vi "Database.SimpleWriteStationValues.vi"(8 "error in":errorcluster, 10 "FileName":string, 11 "Data in":T1 {"Variant"."TS"."TV"."minimum" format="%#.3f"; "Variant"."TS"."TV"."maximum" format="%#.3f"; "Variant"."TS"."TP"."value" format="%#.3f"}) -> (0 "error out":errorcluster, 3 "Data out":T1 {"Variant"."TS"."TV"."minimum" format="%#.3f"; "Variant"."TS"."TV"."maximum" format="%#.3f"; "Variant"."TS"."TP"."value" format="%#.3f"})   [LabVIEW 2016]
doc: "Write test results (measurement values) to proda database\n\nWabco 2017 All right reserved\nAuthor: maciej.szupienko@wabco-auto.com"
uses:
  Global/ApplicationGlobal.vi
  Database.Main.Data.Sets.ctl
  Database.Main.Data.Status.ctl
  ProdaNG/Controls/ProdaNG.ProcessResult.ctl
  ProdaNG/Controls/ProdaNG.ProcessStepResult.ctl
  ProdaNG/Controls/ProdaNG.TestStepResult.ctl
  ProdaNG/Controls/ProdaNG.TestValueResult.ctl
  ProdaNG/Controls/ProdaNG.Identification.ctl
  Database.Main.Data.ctl
  Database.Main.Data.Results.ctl
  ProdaNG/Controls/ProdaNG.TestStepParam.ctl
  ProdaNG/Controls/ProdaNG.TestValue.ctl
  ProdaNG/Controls/ProdaNG.TestStep.ctl
  ProdaNG/Controls/ProdaNG.ProcessStepParam.ctl
  Database.Main.Data.Variant.ctl
panel:
  out "Prod saved":bool
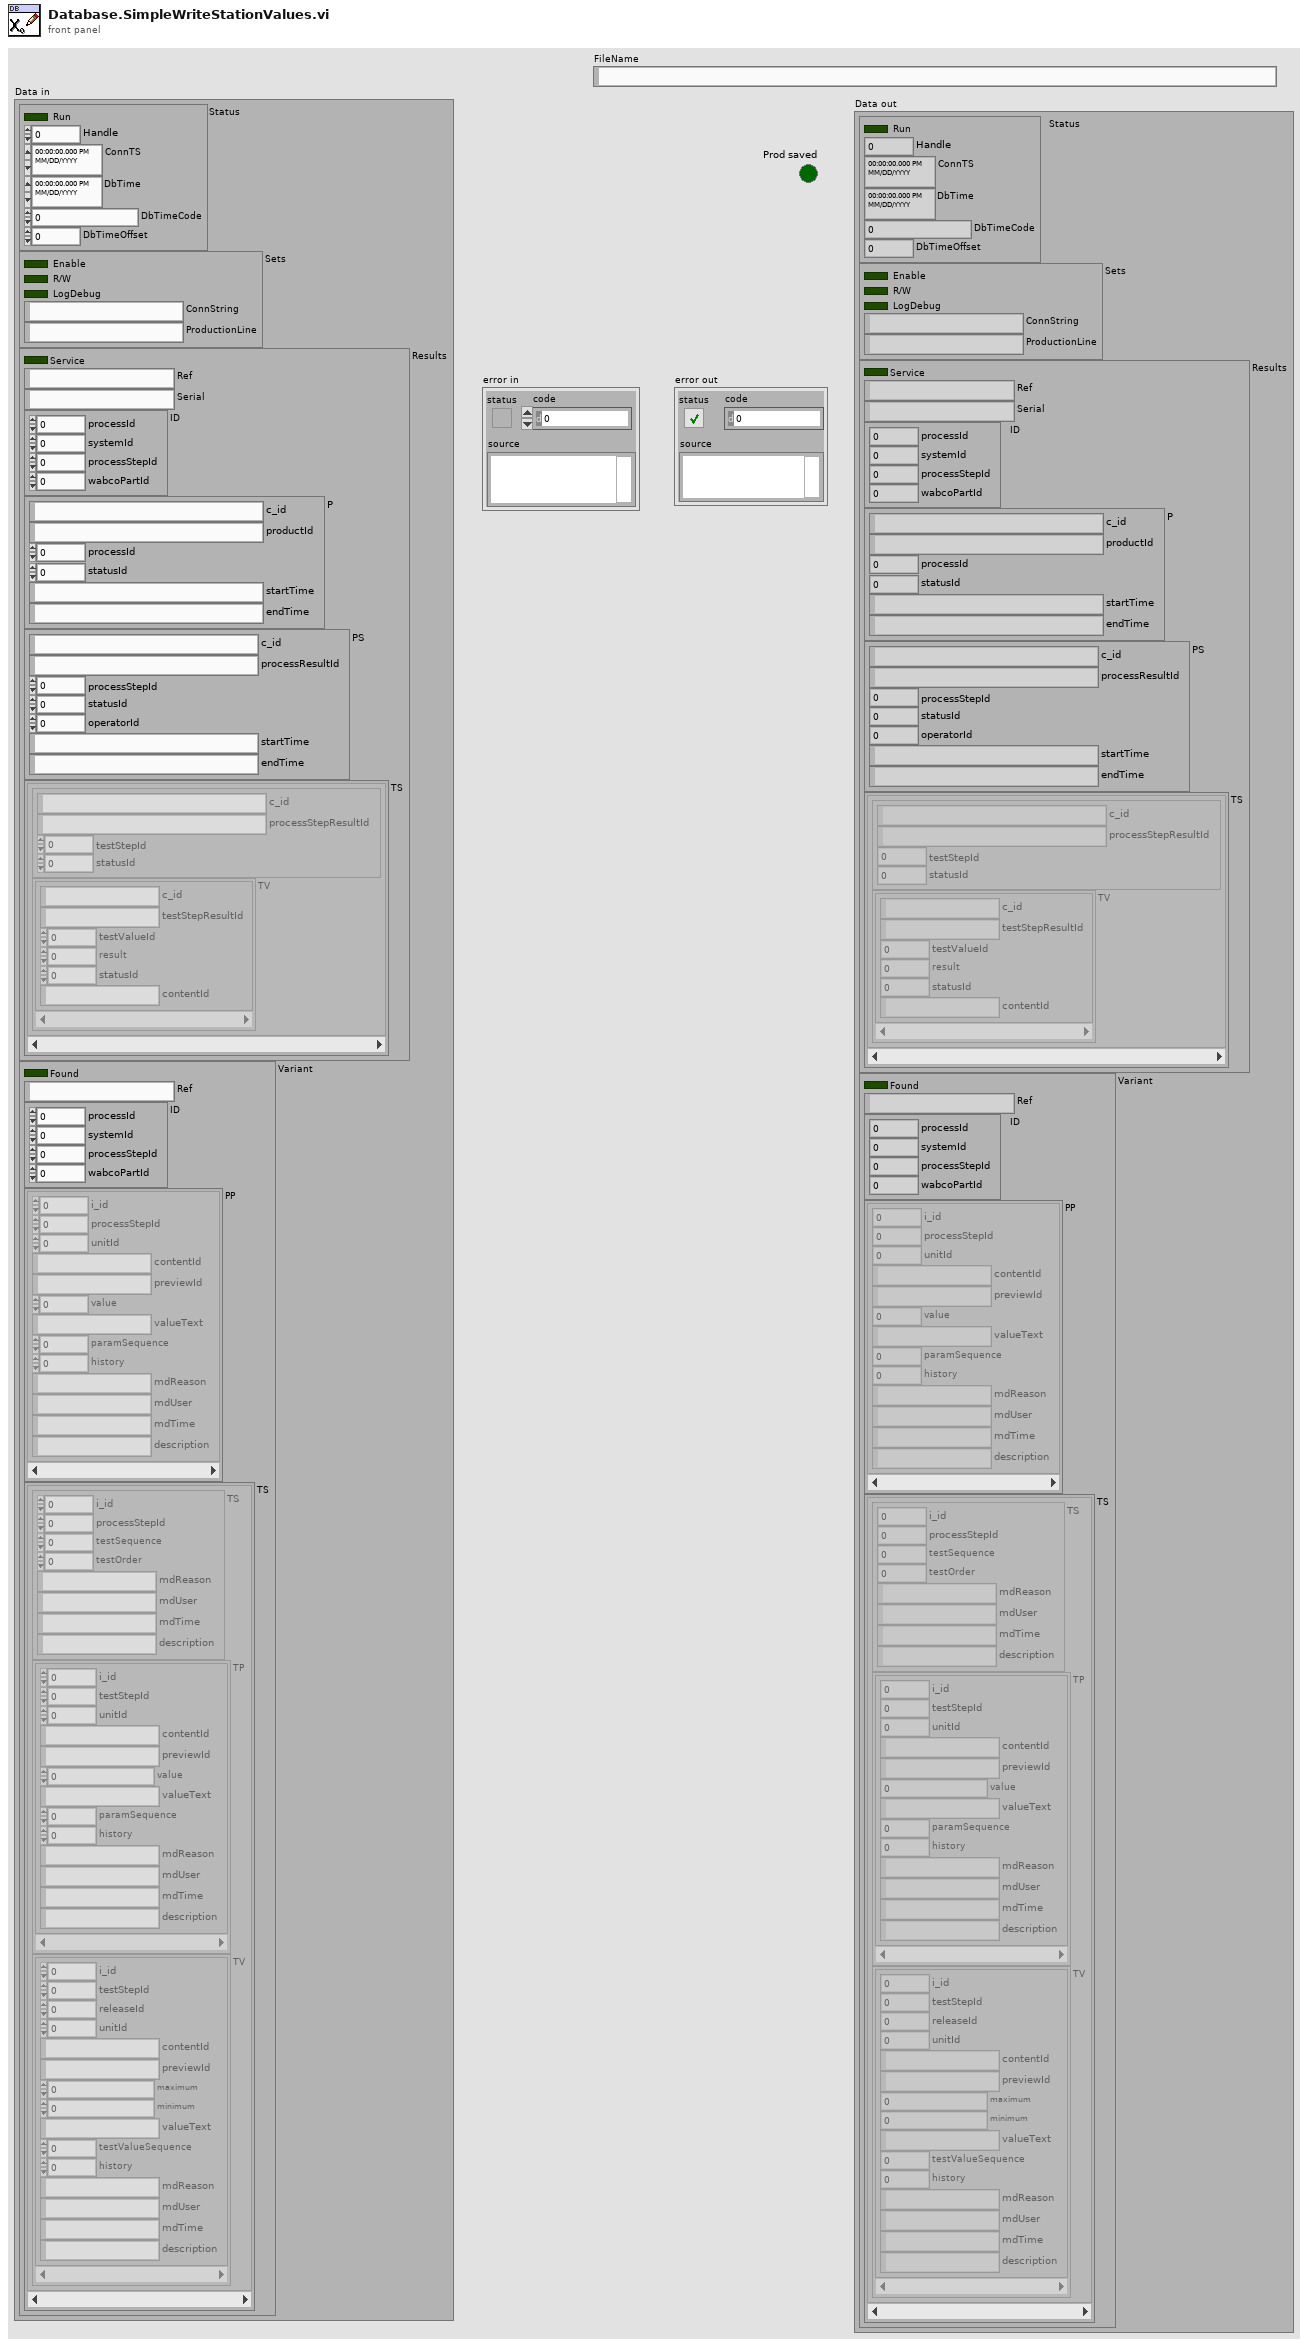
[diagram p1: front panel]
types:
  T1 = typedef "Database.Main.Data.ctl" = cluster{"Status":T2, "Sets":T3, "Results":T4, "Variant":T10}
  T2 = typedef "Database.Main.Data.Status.ctl" = cluster{"Run":bool, "Handle":i32, "ConnTS":timestamp, "DbTime":timestamp, "DbTimeCode":dbl, "DbTimeOffset":dbl}
  T3 = typedef "Database.Main.Data.Sets.ctl" = cluster{"Enable":bool, "R/W":bool, "LogDebug":bool, "ConnString":string, "ProductionLine":string}
  T4 = typedef "Database.Main.Data.Results.ctl" = cluster{"Service":bool, "Ref":string, "Serial":string, "ID":T5, "P":T6, "PS":T7, "TS":cluster{"TS":T8, "TV":T9[]}[]}
  T5 = typedef "ProdaNG.Identification.ctl" = cluster{"processId":i32, "systemId":i32, "processStepId":i32, "wabcoPartId":i32}
  T6 = typedef "ProdaNG.ProcessResult.ctl" = cluster{"c_id":string, "productId":string, "processId":i32, "statusId":i32, "startTime":string, "endTime":string}
  T7 = typedef "ProdaNG.ProcessStepResult.ctl" = cluster{"c_id":string, "processResultId":string, "processStepId":i32, "statusId":i32, "operatorId":i32, "startTime":string, "endTime":string}
  T8 = typedef "ProdaNG.TestStepResult.ctl" = cluster{"c_id":string, "processStepResultId":string, "testStepId":i32, "statusId":i32}
  T9 = typedef "ProdaNG.TestValueResult.ctl" = cluster{"c_id":string, "testStepResultId":string, "testValueId":i32, "result":dbl, "statusId":i32, "contentId":string}
  T10 = typedef "Database.Main.Data.Variant.ctl" = cluster{"Found":bool, "Ref":string, "ID":T5, "PP":T11[], "TS":cluster{"TS":T12, "TP":T13[], "TV":T14[]}[]}
  T11 = typedef "ProdaNG.ProcessStepParam.ctl" = cluster{"i_id":i32, "processStepId":i32, "unitId":i32, "contentId":string, "previewId":string, "value":dbl, "valueText":string, "paramSequence":i32, "history":i32, "mdReason":string, "mdUser":string, "mdTime":string, "description":string}
  T12 = typedef "ProdaNG.TestStep.ctl" = cluster{"i_id":i32, "processStepId":i32, "testSequence":i32, "testOrder":i32, "mdReason":string, "mdUser":string, "mdTime":string, "description":string}
  T13 = typedef "ProdaNG.TestStepParam.ctl" = cluster{"i_id":i32, "testStepId":i32, "unitId":i32, "contentId":string, "previewId":string, "value":dbl, "valueText":string, "paramSequence":i32, "history":i32, "mdReason":string, "mdUser":string, "mdTime":string, "description":string}
  T14 = typedef "ProdaNG.TestValue.ctl" = cluster{"i_id":i32, "testStepId":i32, "releaseId":i32, "unitId":i32, "contentId":string, "previewId":string, "maximum":dbl, "minimum":dbl, "valueText":string, "testValueSequence":i32, "history":i32, "mdReason":string, "mdUser":string, "mdTime":string, "description":string}
  T15 = typedef "ProdaNG.Product.ctl" = cluster{"c_id":string, "wabcoPartId":i32, "serialNumber":string, "comment":string, "individual":i32, "crProcessStepId":i32, "mdProcessStepId":i32, "crTime":string, "mdTime":string}
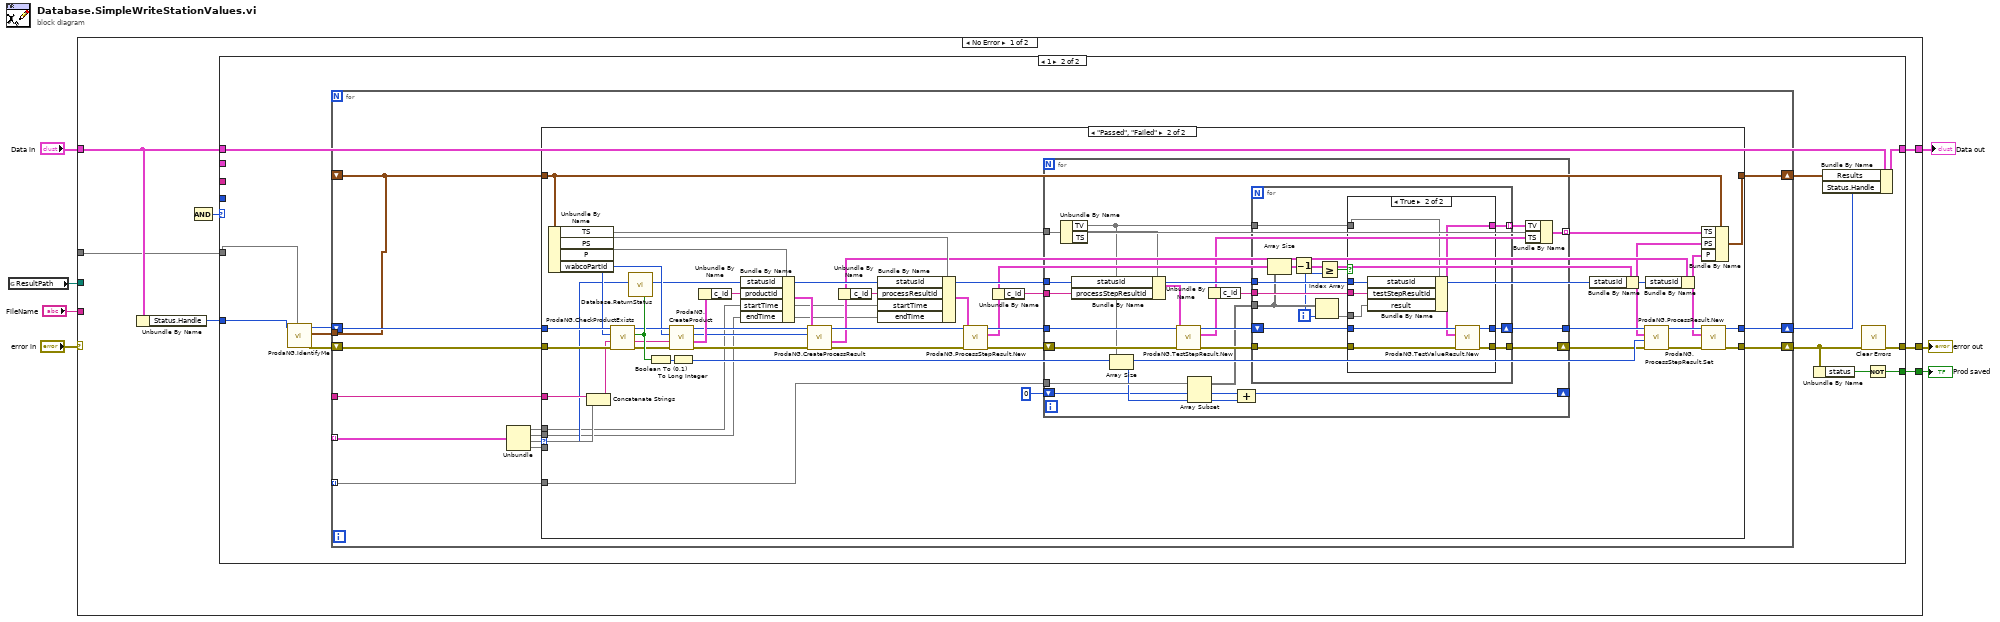
[diagram p0: block diagram]
diagram:
  n1 = global read "ApplicationGlobal.vi" "ResultPath"() -> (w3:path)
  n2 = case shown="No Error" "error in" {
    selector: "error in" -> [_ w146]
    tunnel: [w15 w146] -> w8
    tunnel: "Data in" -> [w11 w145]
    tunnel: [w16 w145] -> w5
    tunnel: [w14 _] -> w4
    tunnel: w3 -> [_ _]
    tunnel: "FileName" -> [_ _]
    tunnel: [w9 _] -> w1
    frame No Error {
      n3 = Unbundle By Name(w11) -> ("Status.Handle"=w10:i32)
      n4 = Compound Arithmetic op=AND() -> (w13:i32)  [unwired: 2 in]
      n5 = case shown="1" w13 {
        tunnel: [_ w36] -> w12
        tunnel: [_ w35] -> w17
        tunnel: w11 -> [w18 w34]
        tunnel: [w18 w33] -> w16
        tunnel: _ -> [_ w32]
        tunnel: [w19 w26] -> w15
        tunnel: [_ w27] -> w14
        tunnel: w10 -> [_ w23]
        tunnel: w9 -> [_ w22]
        frame 0, Default {
        }
        frame 1 {
          n6 = call "ProdaNG.IdentifyMe.vi"("systemName"=w22, "dbHandleIn"=w23) -> ("error out"=w21:errorcluster, "Identification"=w20:T5, "dbHandle"=w24:i32)  [unwired: 7 in]
          n7 = for {
            shift-right: [w45] -> w29
            shift-left: w21 -> [w49]
            shift-right: [w46] -> w30
            shift-left: w24 -> [w48]
            shift-right: [w47] -> w31
            shift-left: [w37] -> _
            tunnel: [w43] -> w25
            tunnel: _ -> [w44] mode=indexing
            tunnel: _ -> [w42] mode=indexing
            tunnel: w20 -> [w37]
            n8 = Unbundle(w44) -> ("date/time string"=w39, "date/time string"=w40, "StatusB"=w38, "SerialB"=w41)
            n9 = case shown="\"Passed\", \"Failed\"" w38 {
              selector: w38 -> [_ w57]
              tunnel: w49 -> [w52 w77]
              tunnel: w48 -> [w51 w76]
              tunnel: [w50 w67] -> w47
              tunnel: [w51 w63] -> w46
              tunnel: w37 -> [w50 w62]
              tunnel: [w52 w61] -> w45
              tunnel: w43 -> [_ w59]
              tunnel: w41 -> [_ w58]
              tunnel: w42 -> [_ w56]
              tunnel: w40 -> [_ w54]
              tunnel: w39 -> [_ w55]
              frame Default {
              }
              frame "Passed", "Failed" {
                n10 = Unbundle By Name(w62) -> ("TS"=w74, "PS"=w73, "P"=w72, "wabcoPartId"=w71:i32)
                n11 = Concatenate Strings(w59, w58) -> (w53:string)
                n12 = call "ProdaNG.CheckProductExists.vi"("error in (no error)"=w77, "serialNumber"=w53, "ID"=w71, "dbHandle"=w76) -> ("error out"=w79:errorcluster, "Results exist?"=w97:bool, "dbHandle out"=w75:i32)  [unwired: 2 in, 3 out]
                n13 = call "Database.ReturnStatus.vi"("repeat"=w97, "Status"=w57) -> ("Step.statusId"=w70:i32)  [unwired: 8 in, 1 out]
                n14 = Boolean To (0,1)(Boolean=w97) -> (0, 1=w78:i16)
                n15 = call "ProdaNG.CreateProduct.vi"("error in (no error)"=w79, "serialNumber"=w53, "ID"=w71, "dbHandle"=w75) -> ("error out"=w91:errorcluster, "Product out"=w96:T15, "dbHandle out"=w92:i32)  [unwired: 4 in, 1 out]
                n16 = To Long Integer(number=w78) -> (32bit integer=w95:i32)
                n17 = Unbundle By Name(w96) -> ("c_id"=w82:string)
                n18 = Bundle By Name(cluster=w72, "statusId"=w70, "productId"=w82, "startTime"=w55, "endTime"=w54) -> (w90:cluster{})
                n19 = call "ProdaNG.CreateProcessResult.vi"("error in (no error)"=w91, "ProcessResult"=w90, "ID"=w71, "dbHandle"=w92) -> ("error out"=w93:errorcluster, "ProcessResult 2"=w68:T6, "dbHandle out"=w94:i32)  [unwired: 5 in]
                n20 = Unbundle By Name(w68) -> ("c_id"=w83:string)
                n21 = Bundle By Name(cluster=w73, "statusId"=w70, "processResultId"=w83, "startTime"=w55, "endTime"=w54) -> (w89:cluster{})
                n22 = call "ProdaNG.ProcessStepResult.New.vi"("error in (no error)"=w93, "ProcessStepResult"=w89, "dbHandle"=w94) -> ("error out"=w81:errorcluster, "ProcessStepResult out"=w65:T7, "dbHandle"=w80:i32)  [unwired: 6 in]
                n23 = Unbundle By Name(w65) -> ("c_id"=w84:string)
                n24 = for {
                  tunnel: [w117] -> w86
                  tunnel: w84 -> [w115]
                  tunnel: w80 -> [w113]
                  tunnel: w56 -> [w103]
                  tunnel: w74 -> [w108]
                  tunnel: w70 -> [w109]
                  tunnel: [w104] -> w69 mode=indexing
                  shift-right: [w116] -> w85
                  shift-left: w81 -> [w114]
                  shift-right: [w98] -> _
                  shift-left: 0 -> [w100]
                  n25 = Unbundle By Name(w108) -> ("TV"=w102, "TS"=w106)
                  n26 = Bundle By Name(cluster=w106, "statusId"=w109, "processStepResultId"=w115) -> (w118:cluster{})
                  n27 = Array Size(array=w102) -> (size(s)=w101:i32)
                  n28 = call "ProdaNG.TestStepResult.New.vi"("error in (no error)"=w114, "TestStepResult"=w118, "dbHandle"=w113) -> ("error out"=w110:errorcluster, "TestStepResult out"=w105:T8, "dbHandle"=w111:i32)  [unwired: 6 in]
                  n29 = Array Subset(array=w103, index=w100, length=w101) -> (w99:void[])
                  n30 = Unbundle By Name(w105) -> ("c_id"=w112:string)
                  n31 = Compound Arithmetic op=ADD(w100, w101) -> (w98:i32)
                  n32 = for "results" {
                    tunnel: w110 -> [w132]
                    tunnel: [w129] -> w116
                    tunnel: w112 -> [w130]
                    shift-right: [w128] -> w117
                    shift-left: w111 -> [w131]
                    tunnel: w99 -> [w123]
                    tunnel: w109 -> [w127]
                    tunnel: w102 -> [w126]
                    tunnel: [w125] -> w107 mode=indexing
                    i -> [w121]
                    n33 = Array Size(array=w123) -> (size(s)=w120:i32)
                    n34 = Decrement(x=w120) -> (x-1=w119:i32)
                    n35 = Index Array(array=w123, index=w121) -> (element=w124)
                    n36 = Greater Or Equal?(x=w119, y=w121) -> (x >= y?=w122:bool)
                    n37 = case shown="True" w122 {
                      tunnel: w132 -> [w134 w144]
                      tunnel: w131 -> [w133 w143]
                      tunnel: w130 -> [_ w142]
                      tunnel: [w134 w141] -> w129
                      tunnel: [w133 w140] -> w128
                      tunnel: w127 -> [_ w139]
                      tunnel: w126 -> [w135 w138]
                      tunnel: [w135 w137] -> w125
                      tunnel: w124 -> [_ w136]
                      frame False {
                      }
                      frame True {
                        n38 = Bundle By Name(cluster=w138, "statusId"=w139, "testStepResultId"=w142, "result"=w136) -> (w137:cluster{})
                        n39 = call "ProdaNG.TestValueResult.New.vi"("error in (no error)"=w144, "TestValueResult"=w137, "dbHandle"=w143) -> ("error out"=w141:errorcluster, "dbHandle"=w140:i32)  [unwired: 7 in]
                      }
                    }
                  }
                  n40 = Bundle By Name(cluster=w108, "TV"=w107, "TS"=w105) -> (w104:cluster{})
                }
                n41 = Bundle By Name(cluster=w65, "statusId"=w70) -> (w64:T7)
                n42 = call "ProdaNG.ProcessStepResult.Set.vi"("error in (no error)"=w85, "isRepeat (0)"=w95, "ProcessStepResult"=w64, "dbHandle"=w86) -> ("error out"=w88:errorcluster, "dbHandle"=w87:i32)  [unwired: 6 in]
                n43 = Bundle By Name(cluster=w68, "statusId"=w70) -> (w66:T6)
                n44 = Bundle By Name(cluster=w62, "TS"=w69, "PS"=w64, "P"=w66) -> (w67:T5)
                n45 = call "ProdaNG.ProcessResult.New.vi"("error in (no error)"=w88, "ProcessResult"=w66, "dbHandle"=w87) -> ("error out"=w61:errorcluster, "dbHandle"=w63:i32)  [unwired: 6 in, 1 out]
              }
            }
          }
          n46 = Unbundle By Name(w29) -> ("status"=w28:bool)
          n47 = Bundle By Name(cluster=w34, "Results"=w31, "Status.Handle"=w30) -> (w33:T1)
          n48 = call <vilib>:"Clear Errors.vi"("error in (no error)"=w29) -> ("error out"=w26:errorcluster)  [unwired: 5 in, 1 out]
          n49 = Not(x=w28) -> (.not. x?=w27:bool)
        }
      }
    }
    frame Error {
    }
  }
  "error out" <- w8
  "Prod saved" <- w4
  "Data out" <- w5
